vi "flashLED_DG535andcount.vi"(3 "error in":errorcluster, 7 "GPIB address":string="15", 9 "Period":i64=20, 10 "Counter 2":tag="Dev1/ctr1", 11 "Counter 1":tag="Dev1/ctr0") -> (1 "Counts 2":u32, 2 "Counts 1":u32, 4 "error out":errorcluster)   [LabVIEW 2013]
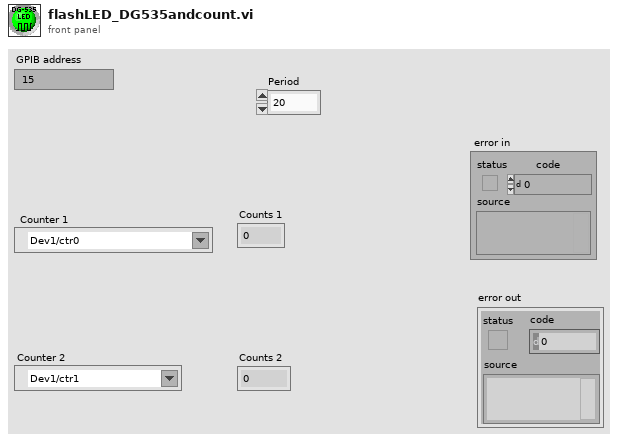
[diagram p1: front panel]
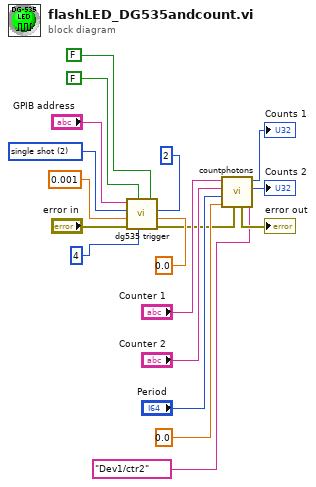
[diagram p0: block diagram]
diagram:
  w10 = u32 2 items=["internal", "external", "single shot", "burst", "line"] ("trigger")
  n1 = call "dg535 trigger.vi"("external trigger level"=sgl 0.0, "burst count"=2, "trigger slope"=FALSE, "burst period"=4, "input impedance"=FALSE, "error in"="error in", "internal/burst trigger rate"=0.001, "trigger"=w10, "GPIB address"="GPIB address") -> ("error out"=w2:errorcluster)
  n2 = call "countphotons.vi"("Gating Counter"=tag "Dev1/ctr2", "error in"=w2, "Initial delay (ms)"=0.0 ("Initial Delay"), "Count time (ms)"="Period", "Input Counter 2"="Counter 2", "Input Counter 1"="Counter 1") -> ("Pulses Counted 2"=→"Counts 2":u32, "Pulses Counted"=→"Counts 1":u32, "error out"=→"error out":errorcluster)  [unwired: 3 in]
